vi "Satisfies.vi"(8 "error in (no error)":errorcluster, 10 "Version Range":string, 11 "Semver in":refnum<class "Semver.lvclass">) -> (0 "error out":errorcluster, 2 "Satisfies?":bool)   [LabVIEW 2017, in "Semver.lvlib" / "Semver.lvclass"]
uses:
  Semver.lvclass
  Semver.lvclass/Semver.ctl
  Parse Number.vi
  <vilib>/Utility/error.llb/Error Cluster From Error Code.vi
  <vilib>/ErrorRing/Error Ring.xnode
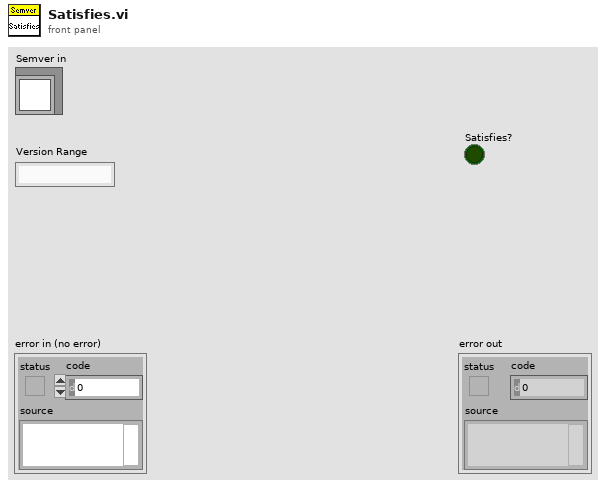
[diagram p1: front panel]
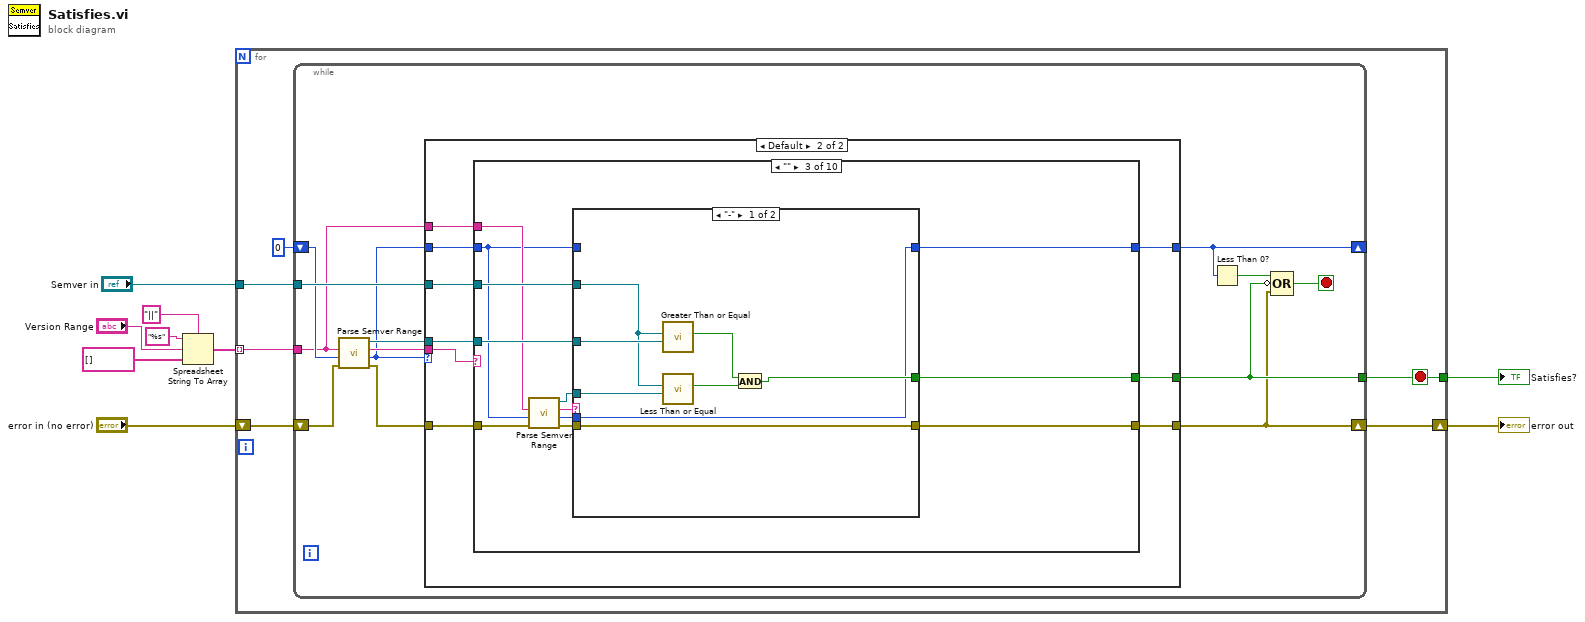
[diagram p0: block diagram]
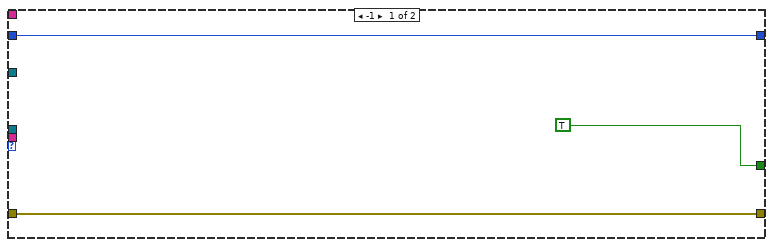
[diagram p2: hidden frame]
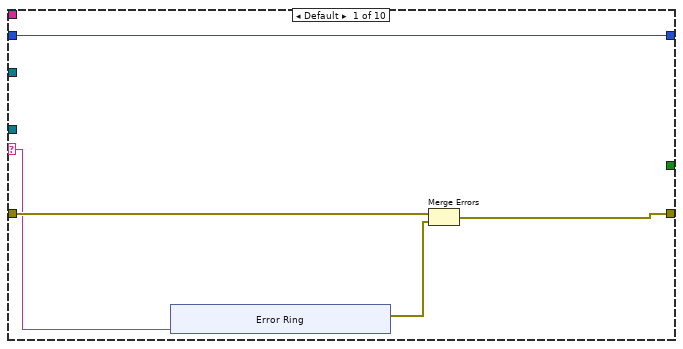
[diagram p3: hidden frame]
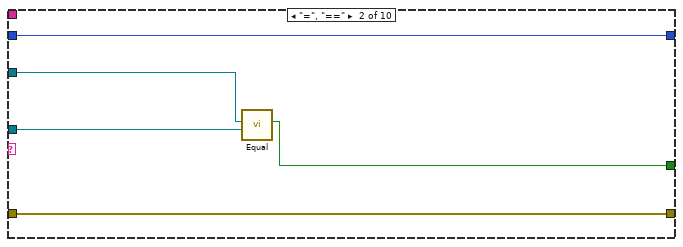
[diagram p4: hidden frame]
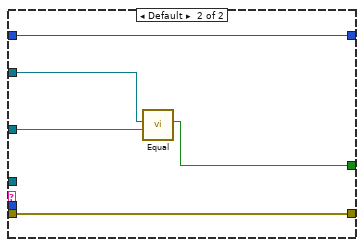
[diagram p5: hidden frame]
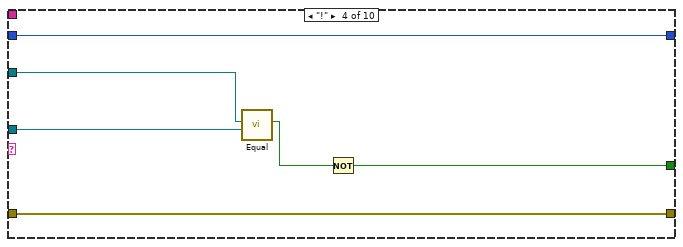
[diagram p6: hidden frame]
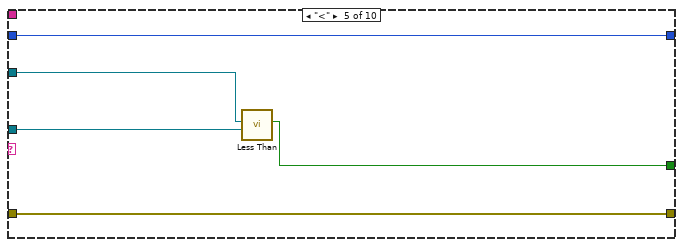
[diagram p7: hidden frame]
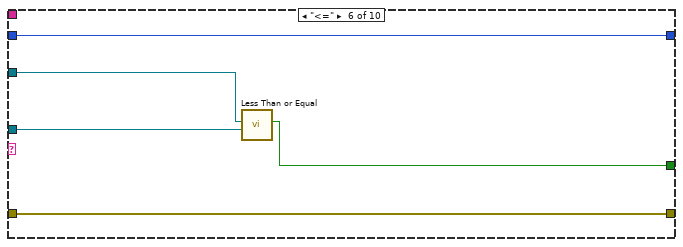
[diagram p8: hidden frame]
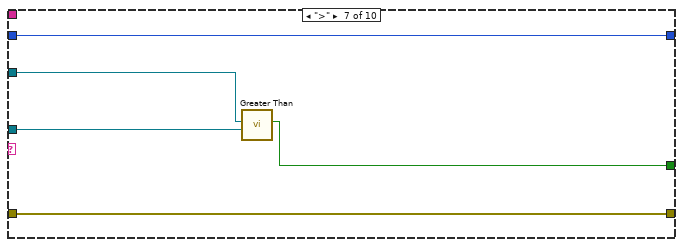
[diagram p9: hidden frame]
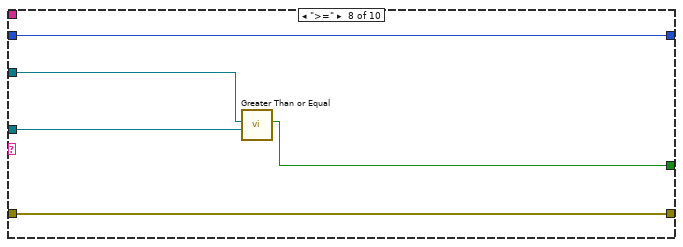
[diagram p10: hidden frame]
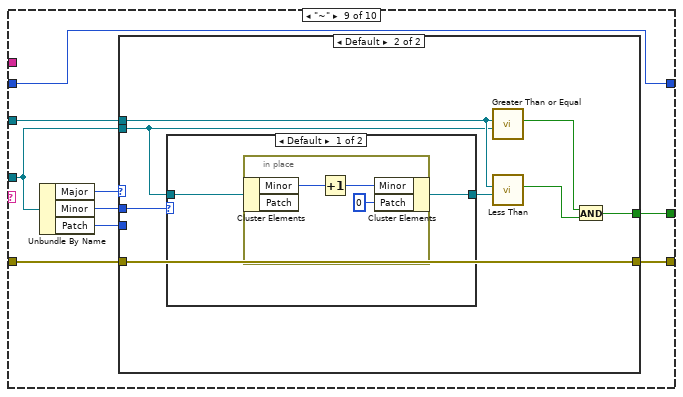
[diagram p11: hidden frame]
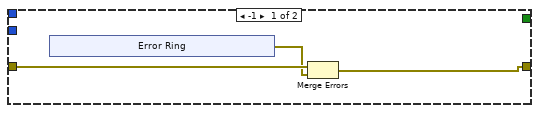
[diagram p12: hidden frame]
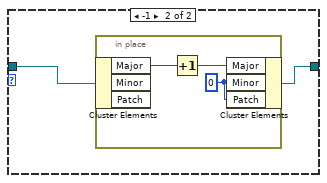
[diagram p13: hidden frame]
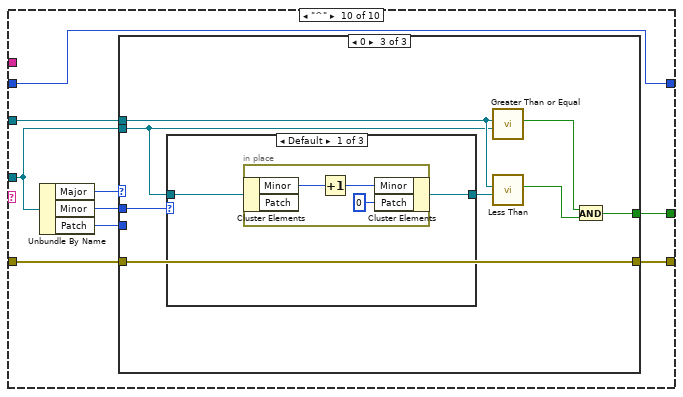
[diagram p14: hidden frame]
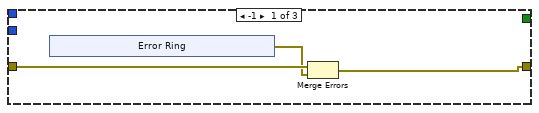
[diagram p15: hidden frame]
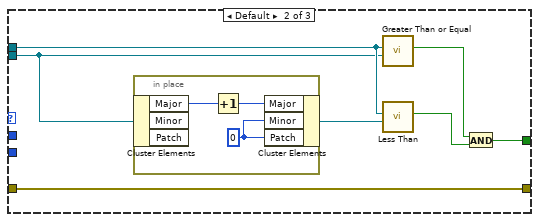
[diagram p16: hidden frame]
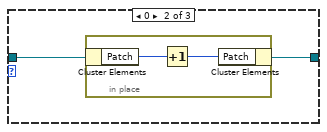
[diagram p17: hidden frame]
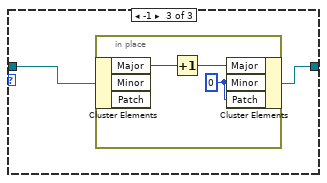
[diagram p18: hidden frame]
diagram:
  n1 = Spreadsheet String To Array(delimiter (Tab)="||", format string="%s", spreadsheet string="Version Range", array type (2D Dbl)=string[] []) -> (array=w3:string[])
  n2 = for {
    shift-right: [w12] -> w8
    shift-left: "error in (no error)" -> [w11]
    tunnel: w3 -> [w13] mode=indexing
    tunnel: "Semver in" -> [w15]
    tunnel: [w14] -> w1
    stop <- w14 stop-if-true
    n3 = while {
      tunnel: w15 -> [w28]
      tunnel: [w20] -> w14
      tunnel: w13 -> [w19]
      shift-right: [w16] -> w12
      shift-left: w11 -> [w25]
      shift-right: [w17] -> _
      shift-left: 0 ("Offset out") -> [w23]
      stop <- w21 stop-if-true
      n4 = call "Parse Semver Range.vi"("error in (no error)"=w25, "Offset in"=w23, "Range Specifier"=w19) -> ("error out"=w24:errorcluster, "Offset out"=w18:i32, "Operator"=w26:string, "Semver out"=w27:refnum<class "Semver.lvclass">)  [unwired: 5 in]
      n5 = case shown="Default" w18 {
        tunnel: w28 -> [_ w40]
        tunnel: [TRUE ("Version 1 >= Version 2") w39] -> w20
        tunnel: w27 -> [_ w38]
        tunnel: w26 -> [_ w37]
        tunnel: [w30 w36] -> w16
        tunnel: w24 -> [w30 w35]
        tunnel: w19 -> [_ w34]
        tunnel: w18 -> [w29 w33]
        tunnel: [w29 w32] -> w17
        frame -1 {
        }
        frame Default {
          n6 = case shown="\"\"" w37 {
            selector: w37 -> [w44 _ _ _ _ _ _ _ _ _]
            tunnel: w40 -> [_ w57 w69 w88 w93 w98 w103 w108 w115 w150]
            tunnel: [_ w55 w67 w84 w91 w96 w101 w106 w116 w151] -> w39
            tunnel: w38 -> [_ w56 w68 w87 w92 w97 w102 w107 w117 w152]
            tunnel: [w43 w54 w64 w85 w90 w95 w100 w105 w113 w148] -> w36
            tunnel: w35 -> [w45 w54 w66 w85 w90 w95 w100 w105 w114 w149]
            tunnel: w34 -> [_ _ w65 _ _ _ _ _ _ _]
            tunnel: w33 -> [w41 w53 w59 w83 w89 w94 w99 w104 w109 w144]
            tunnel: [w41 w53 w60 w83 w89 w94 w99 w104 w109 w144] -> w32
            frame Default {
              n7 = xnode "Error Ring"("parameter 0"=w44) -> ("error out"=w42:errorcluster)
              n8 = Merge Errors(w45, w42) -> (w43:errorcluster)
            }
            frame "=", "==" {
              n9 = call "Equal.vi"("Semver 2"=w56, "Semver 1"=w57) -> ("Version 1 = Version 2"=w55:bool)  [unwired: 9 in]
            }
            frame "" {
              n10 = call "Parse Semver Range.vi"("error in (no error)"=w66, "Offset in"=w59, "Range Specifier"=w65) -> ("error out"=w63:errorcluster, "Offset out"=w58:i32, "Operator"=w62:string, "Semver out"=w61:refnum<class "Semver.lvclass">)  [unwired: 5 in]
              n11 = case shown="\"-\"" w62 {
                tunnel: w69 -> [w75 w82]
                tunnel: w68 -> [w77 w81]
                tunnel: [w71 w80] -> w67
                tunnel: [w76 w79] -> w64
                tunnel: w63 -> [w76 w79]
                tunnel: w61 -> [w74 _]
                tunnel: [w70 w78] -> w60
                tunnel: w59 -> [_ w78]
                tunnel: w58 -> [w70 _]
                frame "-" {
                  n12 = call "Greater Than or Equal.vi"("Semver 2"=w77, "Semver 1"=w75) -> ("Version 1 >= Version 2"=w72:bool)  [unwired: 9 in]
                  n13 = call "Less Than or Equal.vi"("Semver 2"=w74, "Semver 1"=w75) -> ("Version 1 <= Version 2"=w73:bool)  [unwired: 9 in]
                  n14 = And(x=w72, y=w73) -> (x .and. y?=w71:bool)
                }
                frame Default {
                  n15 = call "Equal.vi"("Semver 2"=w81, "Semver 1"=w82) -> ("Version 1 = Version 2"=w80:bool)  [unwired: 9 in]
                }
              }
            }
            frame "!" {
              n16 = call "Equal.vi"("Semver 2"=w87, "Semver 1"=w88) -> ("Version 1 = Version 2"=w86:bool)  [unwired: 9 in]
              n17 = Not(x=w86) -> (.not. x?=w84:bool)
            }
            frame "<" {
              n18 = call "Less Than.vi"("Semver 2"=w92, "Semver 1"=w93) -> ("Version 1 < Version 2"=w91:bool)  [unwired: 9 in]
            }
            frame "<=" {
              n19 = call "Less Than or Equal.vi"("Semver 2"=w97, "Semver 1"=w98) -> ("Version 1 <= Version 2"=w96:bool)  [unwired: 9 in]
            }
            frame ">" {
              n20 = call "Greater Than.vi"("Semver 2"=w102, "Semver 1"=w103) -> ("Version 1 > Version 2"=w101:bool)  [unwired: 9 in]
            }
            frame ">=" {
              n21 = call "Greater Than or Equal.vi"("Semver 2"=w107, "Semver 1"=w108) -> ("Version 1 >= Version 2"=w106:bool)  [unwired: 9 in]
            }
            frame "~" {
              n22 = Unbundle By Name(w117) -> ("Major"=w112:i32, "Minor"=w111:i32, "Patch"=w110:i32)
              n23 = case shown="Default" w112 {
                tunnel: w117 -> [_ w126]
                tunnel: [_ w133] -> w116
                tunnel: w115 -> [_ w131]
                tunnel: w114 -> [w120 w129]
                tunnel: [w119 w129] -> w113
                tunnel: w111 -> [_ w128]
                tunnel: w110 -> [_ _]
                frame -1 {
                  n24 = xnode "Error Ring"() -> ("error out"=w118:errorcluster)
                  n25 = Merge Errors(w120, w118) -> (w119:errorcluster)
                }
                frame Default {
                  n26 = case shown="Default" w128 {
                    tunnel: [w134 w139] -> w127
                    tunnel: w126 -> [w135 w140]
                    frame Default {
                      n27 = in-place {
                        n28 = in-place-cluster #1(w135) -> ("Minor"=w138:i32)  [unwired: 1 out]
                        n29 = Increment(x=w138) -> (x+1=w137:i32)
                        n30 = in-place-cluster #1("Minor"=w137, "Patch"=0) -> (w134:refnum<class "Semver.lvclass">)
                      }
                    }
                    frame -1 {
                      n31 = in-place {
                        w141 = 0 ("Minor")
                        n32 = in-place-cluster #2(w140) -> ("Major"=w143:i32)  [unwired: 2 out]
                        n33 = Increment(x=w143) -> (x+1=w142:i32)
                        n34 = in-place-cluster #2("Major"=w142, "Minor"=w141, "Patch"=w141) -> (w139:refnum<class "Semver.lvclass">)
                      }
                    }
                  }
                  n35 = call "Greater Than or Equal.vi"("Semver 2"=w126, "Semver 1"=w131) -> ("Version 1 >= Version 2"=w132:bool)  [unwired: 9 in]
                  n36 = call "Less Than.vi"("Semver 2"=w127, "Semver 1"=w131) -> ("Version 1 < Version 2"=w130:bool)  [unwired: 9 in]
                  n37 = And(x=w132, y=w130) -> (x .and. y?=w133:bool)
                }
              }
            }
            frame "^" {
              n38 = Unbundle By Name(w152) -> ("Major"=w147:i32, "Minor"=w146:i32, "Patch"=w145:i32)
              n39 = case shown="0" w147 {
                tunnel: w152 -> [_ w161 w171]
                tunnel: [_ w167 w178] -> w151
                tunnel: w150 -> [_ w165 w176]
                tunnel: w149 -> [w155 w163 w174]
                tunnel: [w154 w163 w174] -> w148
                tunnel: w146 -> [_ _ w173]
                tunnel: w145 -> [_ _ _]
                frame -1 {
                  n40 = xnode "Error Ring"() -> ("error out"=w153:errorcluster)
                  n41 = Merge Errors(w155, w153) -> (w154:errorcluster)
                }
                frame Default {
                  n42 = in-place {
                    w168 = 0 ("Patch")
                    n43 = in-place-cluster #3(w161) -> ("Major"=w170:i32)  [unwired: 2 out]
                    n44 = Increment(x=w170) -> (x+1=w169:i32)
                    n45 = in-place-cluster #3("Major"=w169, "Minor"=w168, "Patch"=w168) -> (w162:refnum<class "Semver.lvclass">)
                  }
                  n46 = call "Greater Than or Equal.vi"("Semver 2"=w161, "Semver 1"=w165) -> ("Version 1 >= Version 2"=w166:bool)  [unwired: 9 in]
                  n47 = call "Less Than.vi"("Semver 2"=w162, "Semver 1"=w165) -> ("Version 1 < Version 2"=w164:bool)  [unwired: 9 in]
                  n48 = And(x=w166, y=w164) -> (x .and. y?=w167:bool)
                }
                frame 0 {
                  n49 = case shown="Default" w173 {
                    tunnel: [w179 w184 w188] -> w172
                    tunnel: w171 -> [w180 w185 w189]
                    frame Default {
                      n50 = in-place {
                        n51 = in-place-cluster #4(w180) -> ("Minor"=w183:i32)  [unwired: 1 out]
                        n52 = Increment(x=w183) -> (x+1=w182:i32)
                        n53 = in-place-cluster #4("Minor"=w182, "Patch"=0) -> (w179:refnum<class "Semver.lvclass">)
                      }
                    }
                    frame 0 {
                      n54 = in-place {
                        n55 = in-place-cluster #5(w185) -> ("Patch"=w187:i32)
                        n56 = Increment(x=w187) -> (x+1=w186:i32)
                        n57 = in-place-cluster #5("Patch"=w186) -> (w184:refnum<class "Semver.lvclass">)
                      }
                    }
                    frame -1 {
                      n58 = in-place {
                        w190 = 0 ("Minor")
                        n59 = in-place-cluster #6(w189) -> ("Major"=w192:i32)  [unwired: 2 out]
                        n60 = Increment(x=w192) -> (x+1=w191:i32)
                        n61 = in-place-cluster #6("Major"=w191, "Minor"=w190, "Patch"=w190) -> (w188:refnum<class "Semver.lvclass">)
                      }
                    }
                  }
                  n62 = call "Greater Than or Equal.vi"("Semver 2"=w171, "Semver 1"=w176) -> ("Version 1 >= Version 2"=w177:bool)  [unwired: 9 in]
                  n63 = call "Less Than.vi"("Semver 2"=w172, "Semver 1"=w176) -> ("Version 1 < Version 2"=w175:bool)  [unwired: 9 in]
                  n64 = And(x=w177, y=w175) -> (x .and. y?=w178:bool)
                }
              }
            }
          }
        }
      }
      n65 = Less Than 0?(x=w17) -> (x < 0?=w22:bool)
      n66 = Compound Arithmetic op=OR(w22, invert w20, w16) -> (w21:bool)
    }
  }
  "error out" <- w8
  "Satisfies?" <- w1
